vi "Correct FFid leak Summer 2016.vi"() -> ()   [LabVIEW 2022 SP3]
uses:
  Globals/Meas_global.vi
  <vilib>/Analysis/NI_AALBase.lvlib
  <vilib>/Analysis/baseanly.llb/Mean (DBL).vi
panel:
  in  "Diffusion time":dbl=0.52
  in  "T":dbl=4.16
  in  "K":dbl=0.069
  out "1/x":dbl=0.0025004168056018674
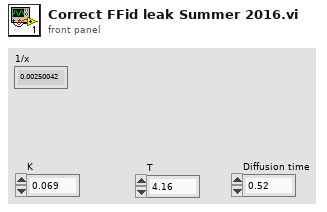
[diagram p1: front panel]
types:
  T1 = typedef "Time_Trace_Cluster.ctl" = cluster{"Weighting":dbl[], "Voltage":dbl[], "Eng Values":dbl[]}
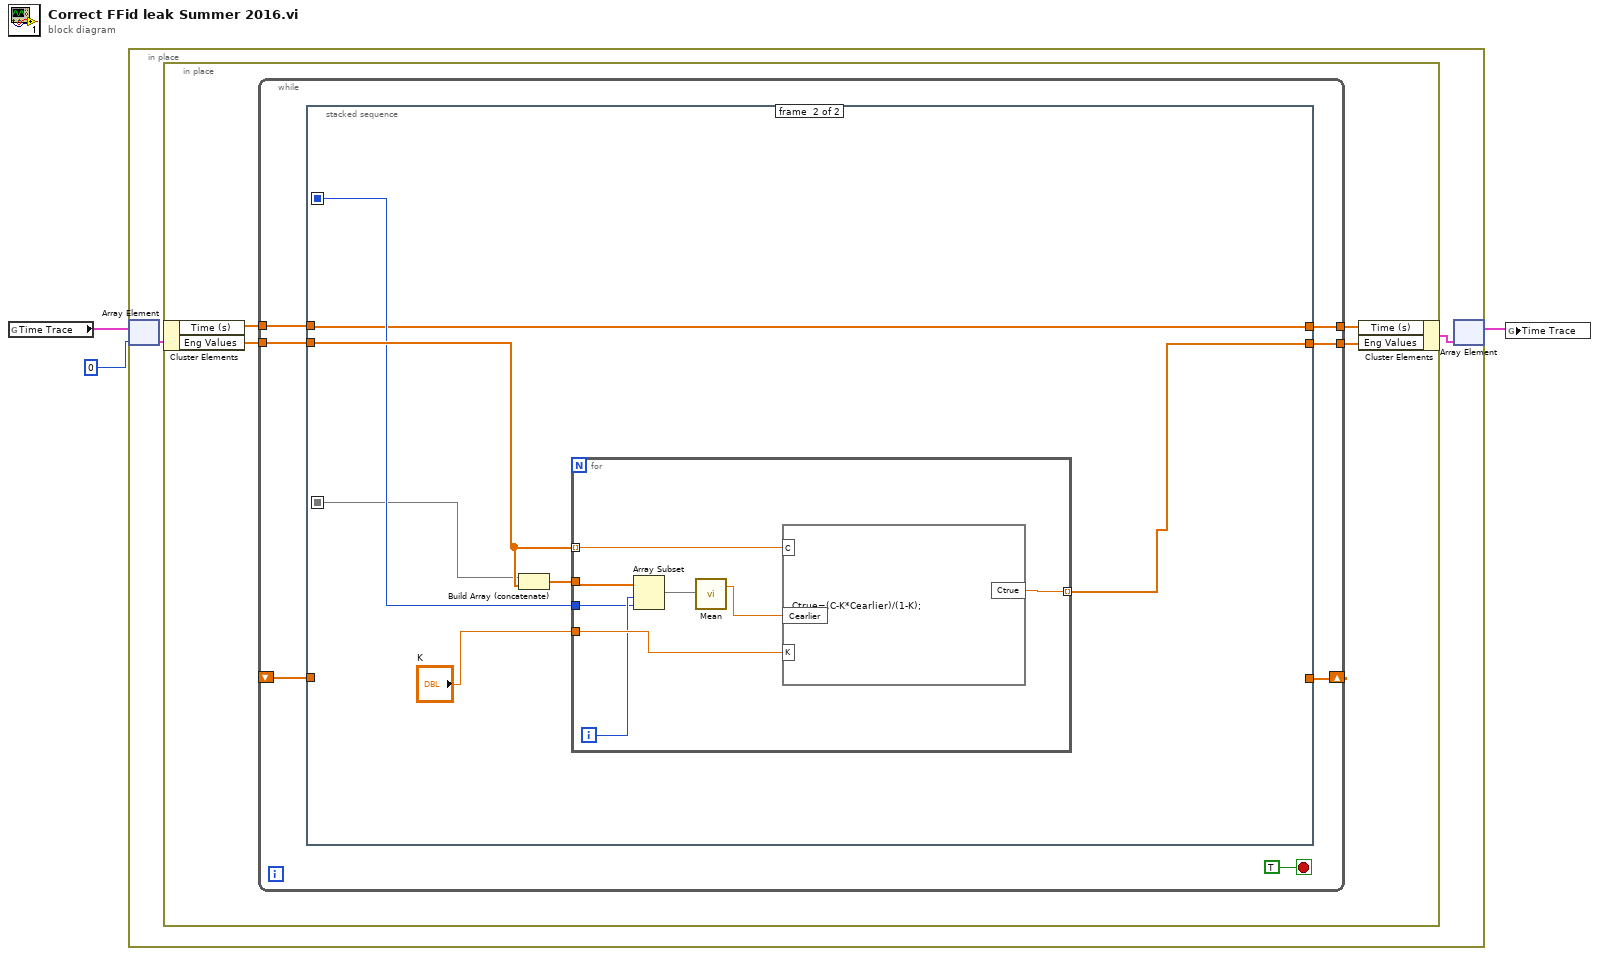
[diagram p0: block diagram]
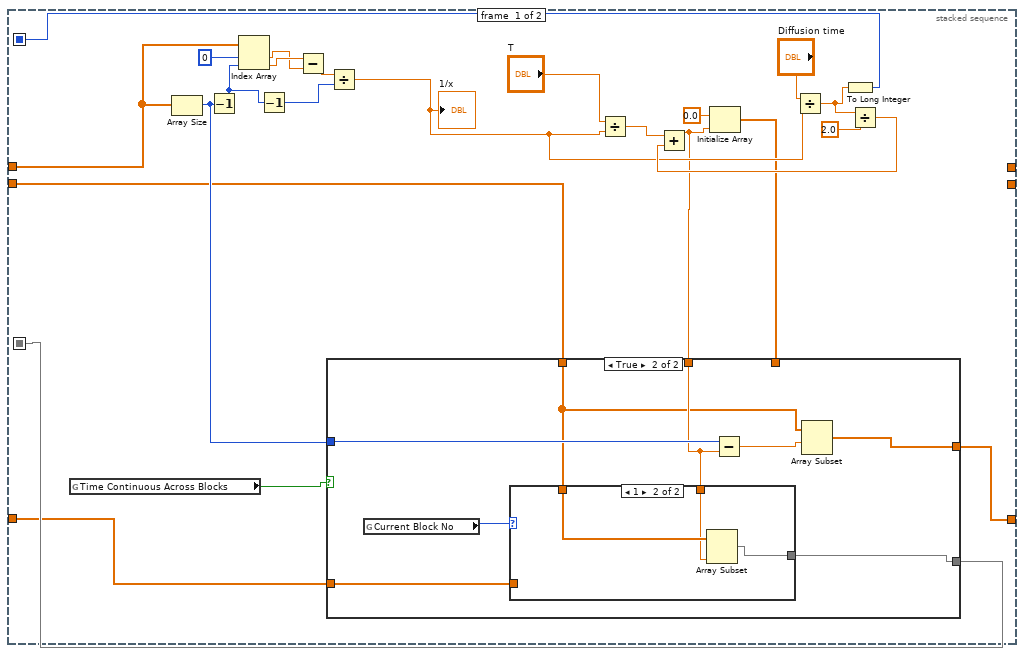
[diagram p2: hidden frame]
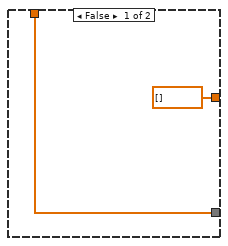
[diagram p3: hidden frame]
diagram:
  n1 = global read "Meas_global.vi" "Time Trace"() -> (w2:T1[])
  n2 = in-place {
    n3 = in-place-array #1(w2, 0) -> (w5:T1)
    n4 = in-place {
      n5 = in-place-cluster #2(w5) -> ("Time (s)"=w9:dbl[], "Eng Values"=w8:dbl[])
      n6 = while {
        tunnel: w9 -> [w16]
        tunnel: w8 -> [w15]
        shift-right: [w12] -> _
        shift-left: _ -> [w13]
        tunnel: [w11] -> w7
        tunnel: [w10] -> w6
        stop <- TRUE stop-if-true
        n7 = stacked-sequence {
          seq-local: [w22 _] -> [_ w55]
          seq-local: [w26 _] -> [_ w58]
          tunnel: w16 -> [w17 w57]
          tunnel: w15 -> [w20 w59]
          tunnel: w13 -> [w19 _]
          tunnel: [w18 _] -> w12
          tunnel: [_ w57] -> w11
          tunnel: [_ w56] -> w10
          frame #0 {
            n8 = global read "Meas_global.vi" "Time Continuous Across Blocks"() -> (w23:bool)
            n9 = Array Size(array=w17) -> (size(s)=w25:i32)
            n10 = Decrement(x=w25) -> (x-1=w32:i32)
            n11 = Index Array(array=w17, index #1=0 ("index"), index #2=w32) -> (element #1=w28:dbl, element #2=w29:dbl)
            n12 = Decrement(x=w32) -> (x-1=w30:i32)
            n13 = Subtract(x=w29, y=w28) -> (x-y=w31:dbl)
            n14 = Divide(x=w31, y=w30) -> (x/y=w27:dbl)
            "1/x" <- w27
            n15 = Divide(x="T", y=w27) -> (x/y=w36:dbl)
            n16 = Divide(x="Diffusion time", y=w27) -> (x/y=w34:dbl)
            n17 = To Long Integer(number=w34) -> (32bit integer=w26:i32)
            n18 = Divide(x=w34, y=2.0) -> (x/y=w35:dbl)
            n19 = Add(x=w36, y=w35) -> (x+y=w24:dbl)
            n20 = Initialize Array(0.0 ("element"), w24) -> (w21:dbl[])
            n21 = case shown="True" w23 {
              tunnel: w25 -> [_ w50]
              tunnel: w24 -> [_ w48]
              tunnel: [w42 w47] -> w22
              tunnel: w21 -> [w42 _]
              tunnel: w20 -> [_ w45]
              tunnel: w19 -> [_ w46]
              tunnel: [dbl[] [] w44] -> w18
              frame False {
              }
              frame True {
                n22 = global read "Meas_global.vi" "Current Block No"() -> (w49:i32)
                n23 = case shown="1" w49 {
                  tunnel: w45 -> [_ w54]
                  tunnel: w48 -> [_ w53]
                  tunnel: [w51 w52] -> w47
                  tunnel: w46 -> [w51 _]
                  frame Default {
                  }
                  frame 1 {
                    n24 = Array Subset(array=w54, length=w53) -> (w52:dbl[])  [unwired: 1 in]
                  }
                }
                n25 = Subtract(x=w50, y=w48) -> (x-y=w43:dbl)
                n26 = Array Subset(array=w45, index=w43) -> (w44:dbl[])  [unwired: 1 in]
              }
            }
          }
          frame #1 {
            n27 = Build Array (concatenate)(w55, w59) -> (w61:dbl[])
            n28 = for {
              tunnel: w59 -> [w68] mode=indexing
              tunnel: w61 -> [w65]
              tunnel: "K" -> [w69]
              tunnel: [w67] -> w56 mode=indexing
              tunnel: w58 -> [w64]
              i -> [w66]
              n29 = Array Subset(array=w65, index=w66, length=w64) -> (w63:dbl[])
              n30 = call-poly <vilib>:"Mean.vi"("X"=w63) -> ("mean"=w62:dbl)  [unwired: 1 out]
              n31 = formula code="Ctrue=(C-K*Cearlier)/(1-K);"("C"=w68, "Cearlier"=w62, "K"=w69) -> ("Ctrue"=w67:dbl)
            }
          }
        }
      }
      n32 = in-place-cluster #2("Time (s)"=w7, "Eng Values"=w6) -> (w4:T1)
    }
    n33 = in-place-array #1(w4) -> (w1:T1[])  [unwired: 1 out]
  }
  n34 = global write "Meas_global.vi" "Time Trace"(w1) -> ()
